vi "LabVIEW_Pad_1.0.vi"() -> ()   [LabVIEW 2016]
panel:
  in  "Nabíjení":bool
  out "Signalizace nabíjení 2":bool
  out "Signalizace prázdné baterie":bool
  out "Signalizace nabíjení":bool
  in  "Clear":bool
  in  "mne/me":bool
  in  "Osoby":bool
  in  "Pady":bool
  in  "SlovniDruhy":bool
  in  "Veta":bool
  in  "Z":bool
  in  "V":bool
  in  "About":bool
  out "Baterie":dbl(slide) scale=1.0..100.0
  in  "S":bool
  in  "P":bool
  in  "M":bool
  in  "L":bool
  in  "F":bool
  in  "B":bool
  in  "icka":bool
  in  "ycka":bool
  in  "Baterie":bool
  out "Display":string
  # "LabVIEW Pad"
  # "LabVIEW"
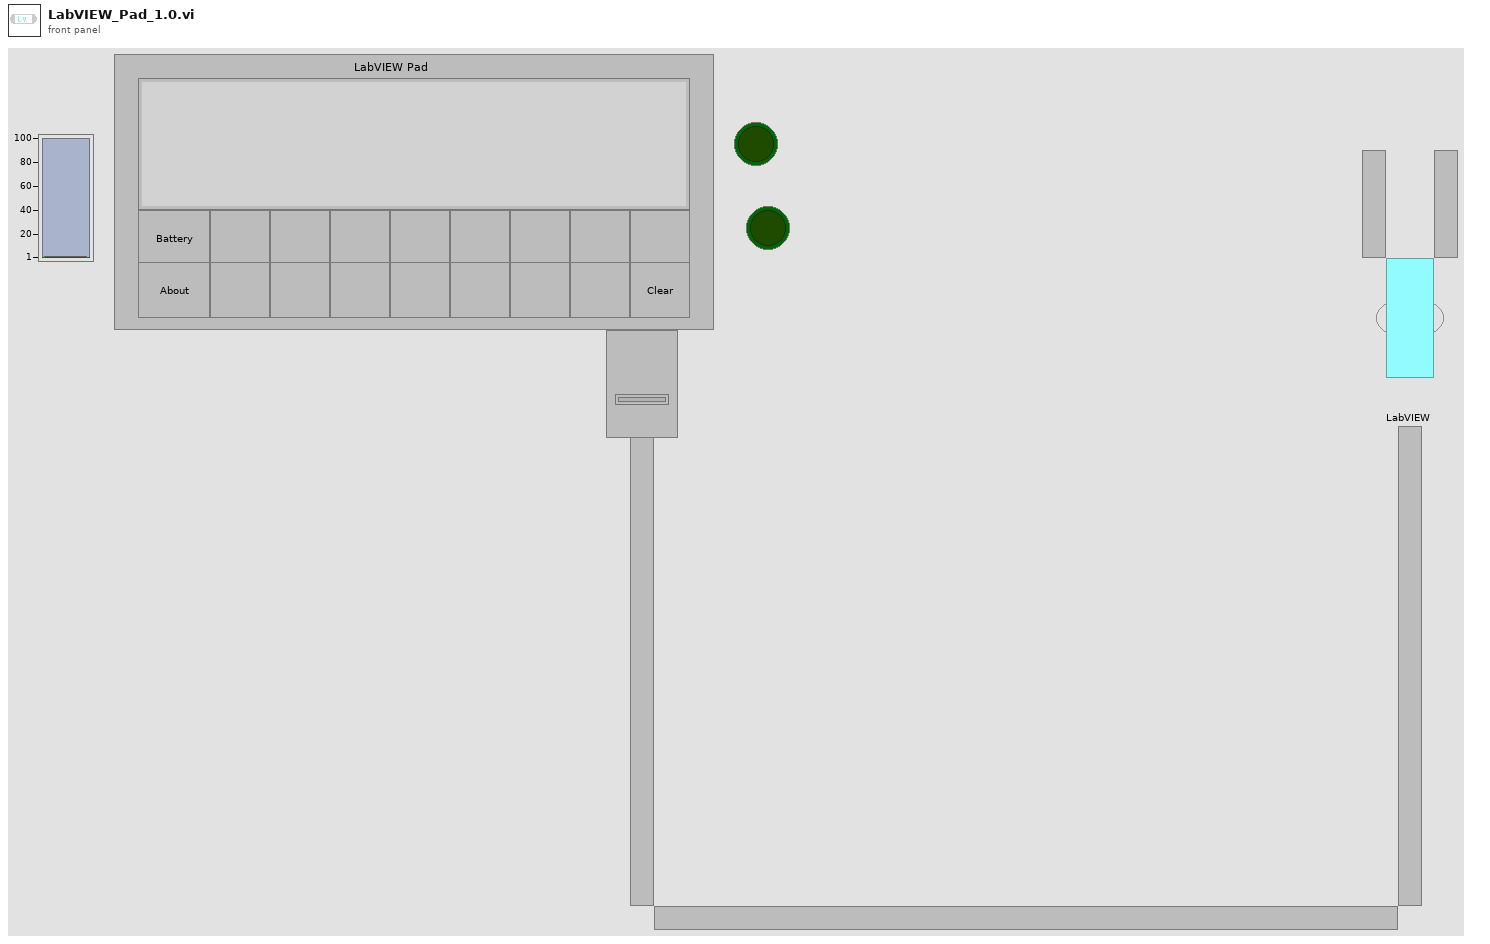
[diagram p1: front panel]
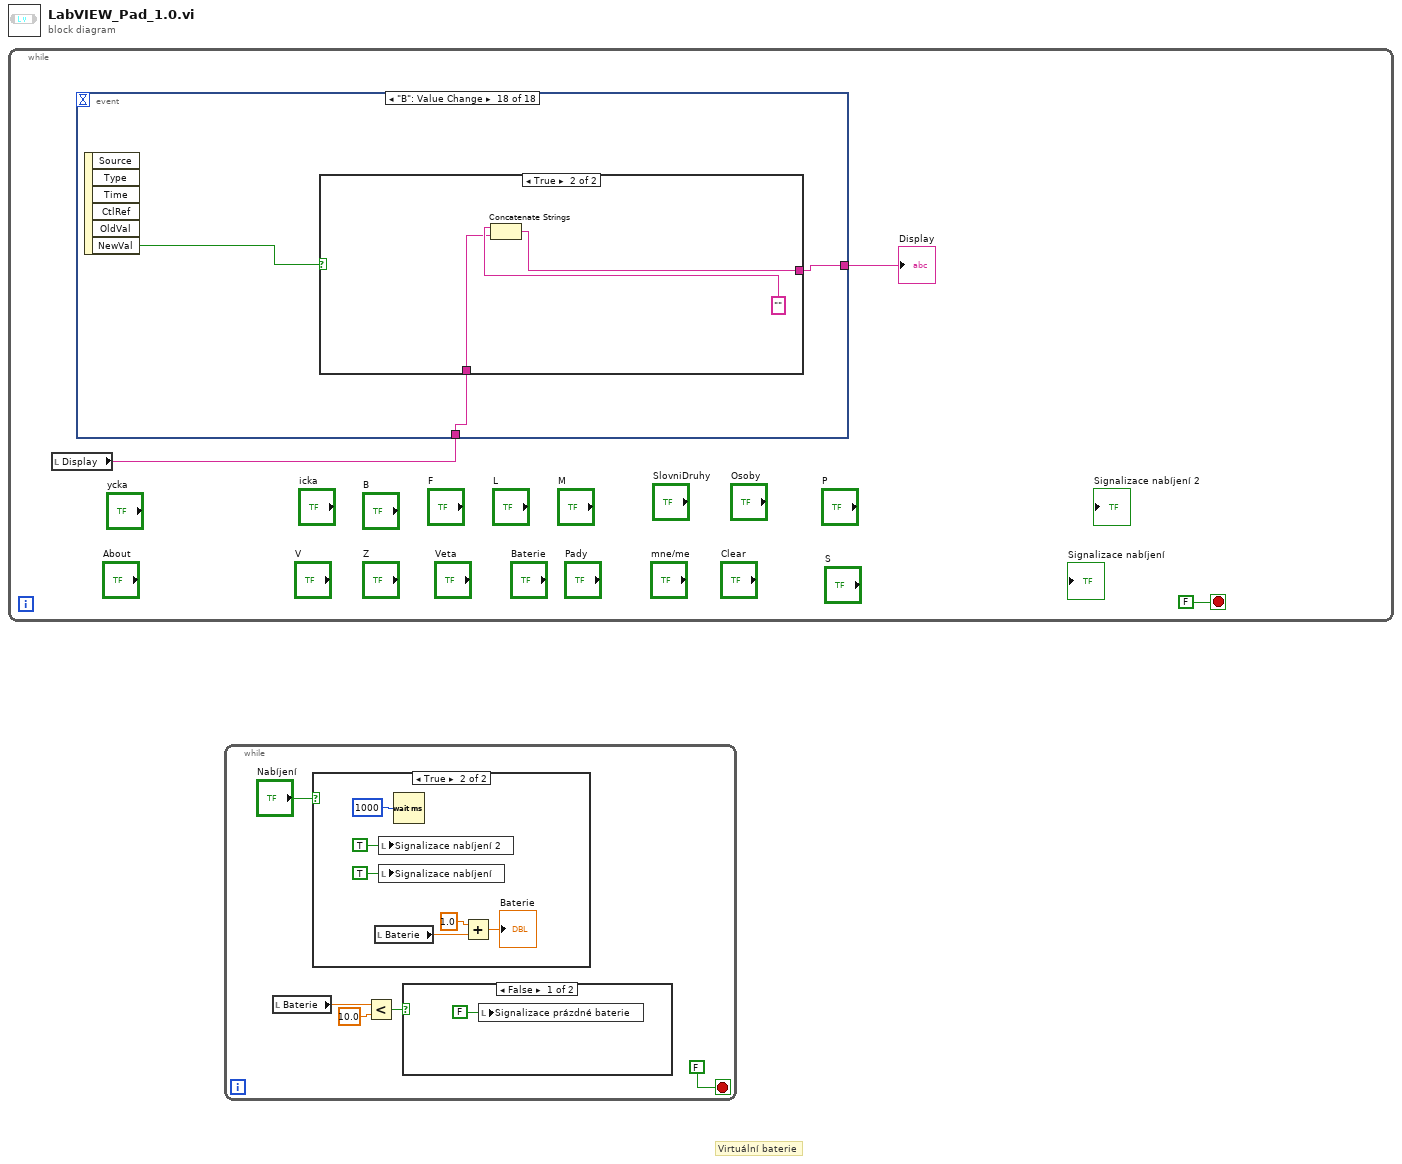
[diagram p0: block diagram]
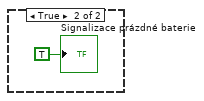
[diagram p2: hidden frame]
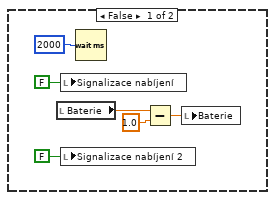
[diagram p3: hidden frame]
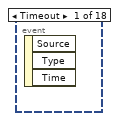
[diagram p4: hidden frame]
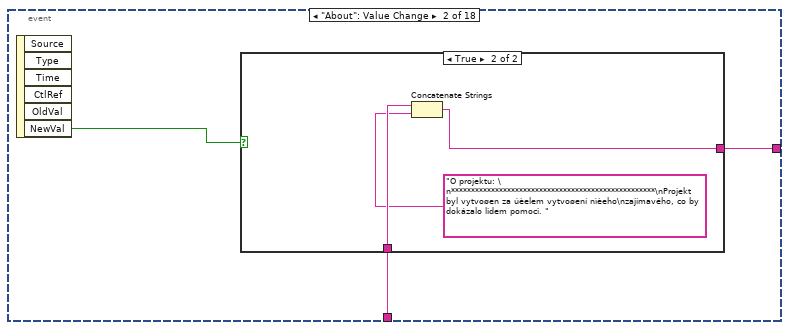
[diagram p5: hidden frame]
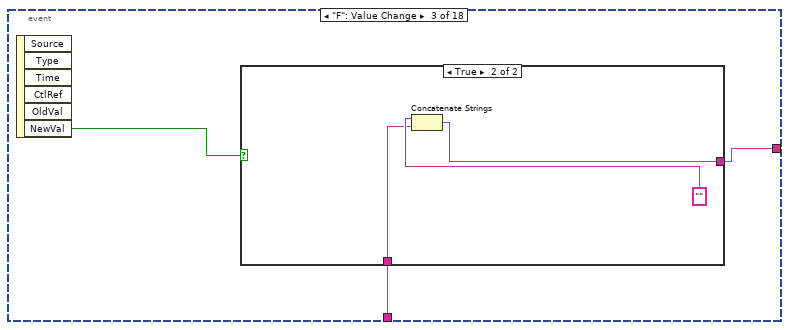
[diagram p7: hidden frame]
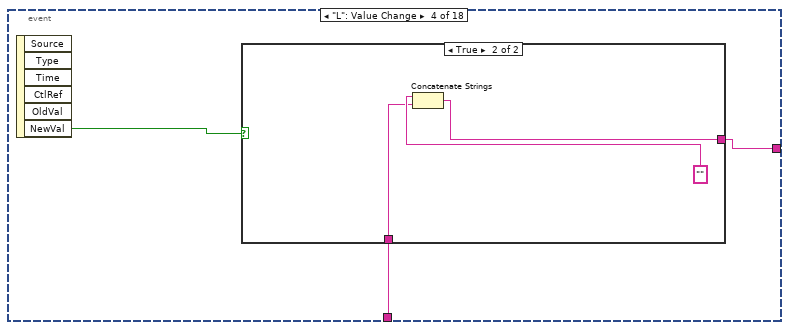
[diagram p9: hidden frame]
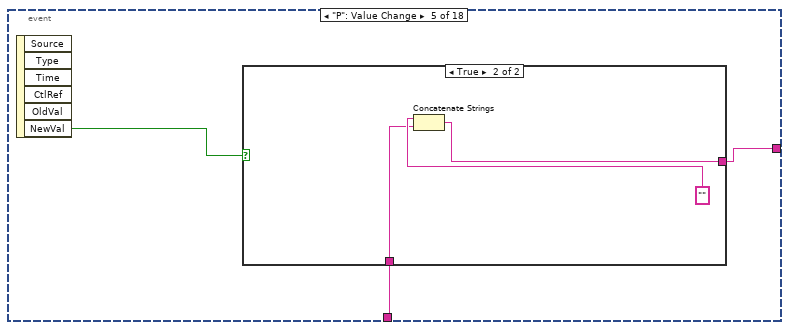
[diagram p11: hidden frame]
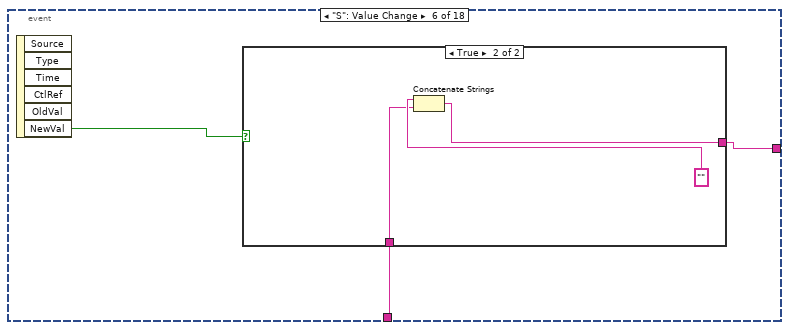
[diagram p13: hidden frame]
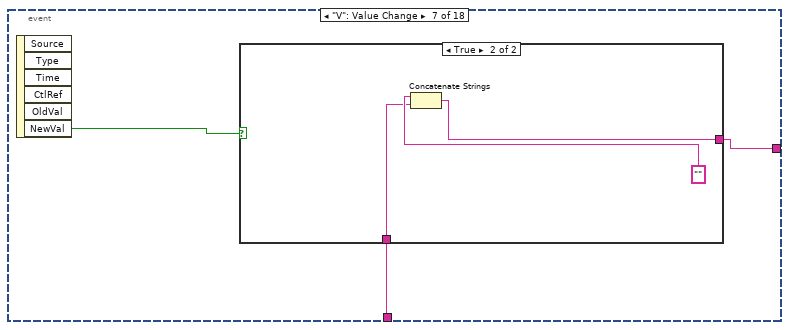
[diagram p15: hidden frame]
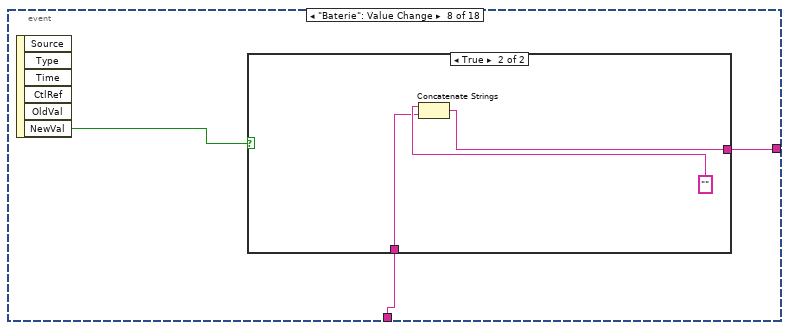
[diagram p17: hidden frame]
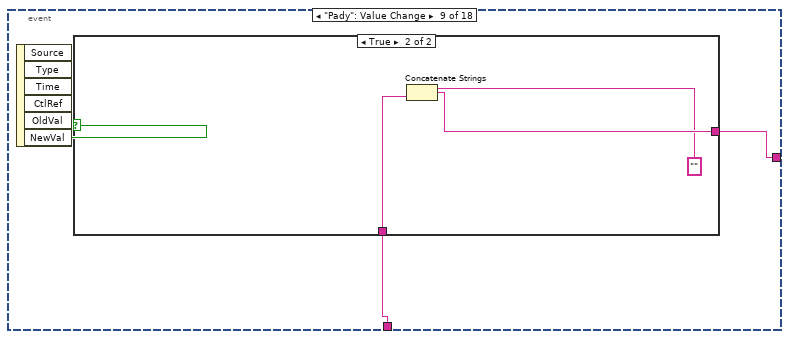
[diagram p19: hidden frame]
diagram:
  # "Virtuální baterie"
  n1 = while {
    stop <- FALSE stop-if-true
    n2 = local read "Display"() -> (w2:string)
    n3 = event shown="[17] \"B\": Value Change" {
      selector: _ -> [_ _ _ _ _ _ _ _ _ _ _ _ _ _ _ _ _ _]
      dyn-events: _ -> [_ _ _ _ _ _ _ _ _ _ _ _ _ _ _ _ _ _]
      timeout: _ -> [_ _ _ _ _ _ _ _ _ _ _ _ _ _ _ _ _ _]
      tunnel: w2 -> [_ w5 w13 w20 w27 w34 w41 w48 w54 w62 w69 w76 w83 w90 w97 w103 _ w112]
      tunnel: [_ w4 w12 w19 w26 w33 w40 w47 w55 w61 w68 w75 w81 w89 w96 w102 _ w110] -> w1
      event Timeout {
        n4 = event-data() -> ()  [unwired: 1 in, 3 out]
      }
      event "About": Value Change {
        n5 = event-data() -> ("NewVal"=w6:bool)  [unwired: 1 in, 5 out]
        n6 = case shown="True" w6 {
          tunnel: w5 -> [w7 w10]
          tunnel: [w7 w8] -> w4
          frame False {
          }
          frame True {
            n7 = Concatenate Strings(w10, "O projektu: \n***************************************************\nProjekt byl vytvoøen za úèelem vytvoøení nìèeho\nzajímavého, co by dokázalo lidem pomoci. " ("string")) -> (w8:string)
          }
        }
      }
      event "F": Value Change {
        n8 = event-data() -> ("NewVal"=w11:bool)  [unwired: 1 in, 5 out]
        n9 = case shown="True" w11 {
          tunnel: w13 -> [w14 w15]
          tunnel: [w14 w17] -> w12
          frame False {
          }
          frame True {
            n10 = Concatenate Strings("" ("string"), w15) -> (w17:string)
          }
        }
      }
      event "L": Value Change {
        n11 = event-data() -> ("NewVal"=w18:bool)  [unwired: 1 in, 5 out]
        n12 = case shown="True" w18 {
          tunnel: w20 -> [w21 w22]
          tunnel: [w21 w24] -> w19
          frame False {
          }
          frame True {
            n13 = Concatenate Strings("" ("string"), w22) -> (w24:string)
          }
        }
      }
      event "P": Value Change {
        n14 = event-data() -> ("NewVal"=w25:bool)  [unwired: 1 in, 5 out]
        n15 = case shown="True" w25 {
          tunnel: w27 -> [w28 w29]
          tunnel: [w28 w31] -> w26
          frame False {
          }
          frame True {
            n16 = Concatenate Strings("" ("string"), w29) -> (w31:string)
          }
        }
      }
      event "S": Value Change {
        n17 = event-data() -> ("NewVal"=w32:bool)  [unwired: 1 in, 5 out]
        n18 = case shown="True" w32 {
          tunnel: w34 -> [w35 w36]
          tunnel: [w35 w38] -> w33
          frame False {
          }
          frame True {
            n19 = Concatenate Strings("" ("string"), w36) -> (w38:string)
          }
        }
      }
      event "V": Value Change {
        n20 = event-data() -> ("NewVal"=w39:bool)  [unwired: 1 in, 5 out]
        n21 = case shown="True" w39 {
          tunnel: w41 -> [w42 w43]
          tunnel: [w42 w45] -> w40
          frame False {
          }
          frame True {
            n22 = Concatenate Strings("" ("string"), w43) -> (w45:string)
          }
        }
      }
      event "Baterie": Value Change {
        n23 = event-data() -> ("NewVal"=w46:bool)  [unwired: 1 in, 5 out]
        n24 = case shown="True" w46 {
          tunnel: w48 -> [w49 w50]
          tunnel: [w49 w52] -> w47
          frame False {
          }
          frame True {
            n25 = Concatenate Strings("" ("string"), w50) -> (w52:string)
          }
        }
      }
      event "Pady": Value Change {
        n26 = event-data() -> ("NewVal"=w53:bool)  [unwired: 1 in, 5 out]
        n27 = case shown="True" w53 {
          tunnel: w54 -> [w56 w57]
          tunnel: [w56 w59] -> w55
          frame False {
          }
          frame True {
            n28 = Concatenate Strings("" ("string"), w57) -> (w59:string)
          }
        }
      }
      event "Osoby": Value Change {
        n29 = event-data() -> ("NewVal"=w60:bool)  [unwired: 1 in, 5 out]
        n30 = case shown="True" w60 {
          tunnel: w62 -> [w63 w64]
          tunnel: [w63 w66] -> w61
          frame False {
          }
          frame True {
            n31 = Concatenate Strings("" ("string"), w64) -> (w66:string)
          }
        }
      }
      event "Veta": Value Change {
        n32 = event-data() -> ("NewVal"=w67:bool)  [unwired: 1 in, 5 out]
        n33 = case shown="True" w67 {
          tunnel: w69 -> [w70 w71]
          tunnel: [w70 w73] -> w68
          frame False {
          }
          frame True {
            n34 = Concatenate Strings("" ("string"), w71) -> (w73:string)
          }
        }
      }
      event "ycka": Value Change {
        n35 = event-data() -> ("NewVal"=w74:bool)  [unwired: 1 in, 5 out]
        n36 = case shown="True" w74 {
          tunnel: w76 -> [w77 w78]
          tunnel: [w77 w80] -> w75
          frame False {
          }
          frame True {
            n37 = Concatenate Strings("" ("string"), w78) -> (w80:string)
          }
        }
      }
      event "icka": Value Change {
        n38 = event-data() -> ("NewVal"=w82:bool)  [unwired: 1 in, 5 out]
        n39 = case shown="True" w82 {
          tunnel: w83 -> [w84 w85]
          tunnel: [w84 w87] -> w81
          frame False {
          }
          frame True {
            n40 = Concatenate Strings("" ("string"), w85) -> (w87:string)
          }
        }
      }
      event "mne/me": Value Change {
        n41 = event-data() -> ("NewVal"=w88:bool)  [unwired: 1 in, 5 out]
        n42 = case shown="True" w88 {
          tunnel: w90 -> [w91 w92]
          tunnel: [w91 w94] -> w89
          frame False {
          }
          frame True {
            n43 = Concatenate Strings("" ("string"), w92) -> (w94:string)
          }
        }
      }
      event "Z": Value Change {
        n44 = event-data() -> ("NewVal"=w95:bool)  [unwired: 1 in, 5 out]
        n45 = case shown="True" w95 {
          tunnel: w97 -> [w98 w99]
          tunnel: [w98 w101] -> w96
          frame False {
          }
          frame True {
            n46 = Concatenate Strings("" ("string"), w99) -> (w101:string)
          }
        }
      }
      event "M": Value Change {
        n47 = event-data() -> ("NewVal"=w104:bool)  [unwired: 1 in, 5 out]
        n48 = case shown="True" w104 {
          tunnel: w103 -> [w105 w106]
          tunnel: [w105 w108] -> w102
          frame False {
          }
          frame True {
            n49 = Concatenate Strings("" ("string"), w106) -> (w108:string)
          }
        }
      }
      event "Clear": Value Change {
        n50 = event-data() -> ()  [unwired: 1 in, 6 out]
        n51 = local write "Display"("" ("Display")) -> ()
      }
      event "B": Value Change {
        n52 = event-data() -> ("NewVal"=w111:bool)  [unwired: 1 in, 5 out]
        n53 = case shown="True" w111 {
          tunnel: w112 -> [w113 w114]
          tunnel: [w113 w116] -> w110
          frame False {
          }
          frame True {
            n54 = Concatenate Strings("" ("string"), w114) -> (w116:string)
          }
        }
      }
    }
    "Display" <- w1
  }
  n55 = while {
    stop <- FALSE stop-if-true
    n56 = local read "Baterie"() -> (w117:dbl)
    n57 = case shown="True" "Nabíjení" {
      frame False {
        n58 = local read "Baterie"() -> (w125:dbl)
        n59 = local write "Signalizace nabíjení"(FALSE ("Signalizace nabíjení")) -> ()
        n60 = local write "Signalizace nabíjení 2"(FALSE ("Signalizace nabíjení 2")) -> ()
        n61 = Wait (ms)(milliseconds to wait=u32 2000) -> ()  [unwired: 1 out]
        n62 = Subtract(x=w125, y=1.0) -> (x-y=w127:dbl)
        n63 = local write "Baterie"(w127) -> ()
      }
      frame True {
        n64 = local read "Baterie"() -> (w130:dbl)
        n65 = local write "Signalizace nabíjení 2"(TRUE ("Signalizace nabíjení 2")) -> ()
        n66 = local write "Signalizace nabíjení"(TRUE ("Signalizace nabíjení")) -> ()
        n67 = Wait (ms)(milliseconds to wait=u32 1000) -> ()  [unwired: 1 out]
        n68 = Add(x=1.0, y=w130) -> (x+y=→"Baterie":dbl)
      }
    }
    n69 = Less?(x=w117, y=10.0) -> (x < y?=w119:bool)
    n70 = case shown="False" w119 {
      frame False {
        n71 = local write "Signalizace prázdné baterie"(FALSE ("Signalizace prázdné baterie")) -> ()
      }
      frame True {
        "Signalizace prázdné baterie" <- TRUE ("Signalizace prázdné baterie")
      }
    }
  }
